vi "260pt Mov Avg.vi"(10 "Value in":dbl) -> (2 "Value out":dbl)   [LabVIEW 2014]
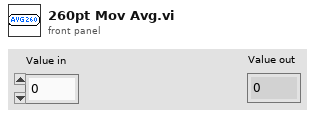
[diagram p1: front panel]
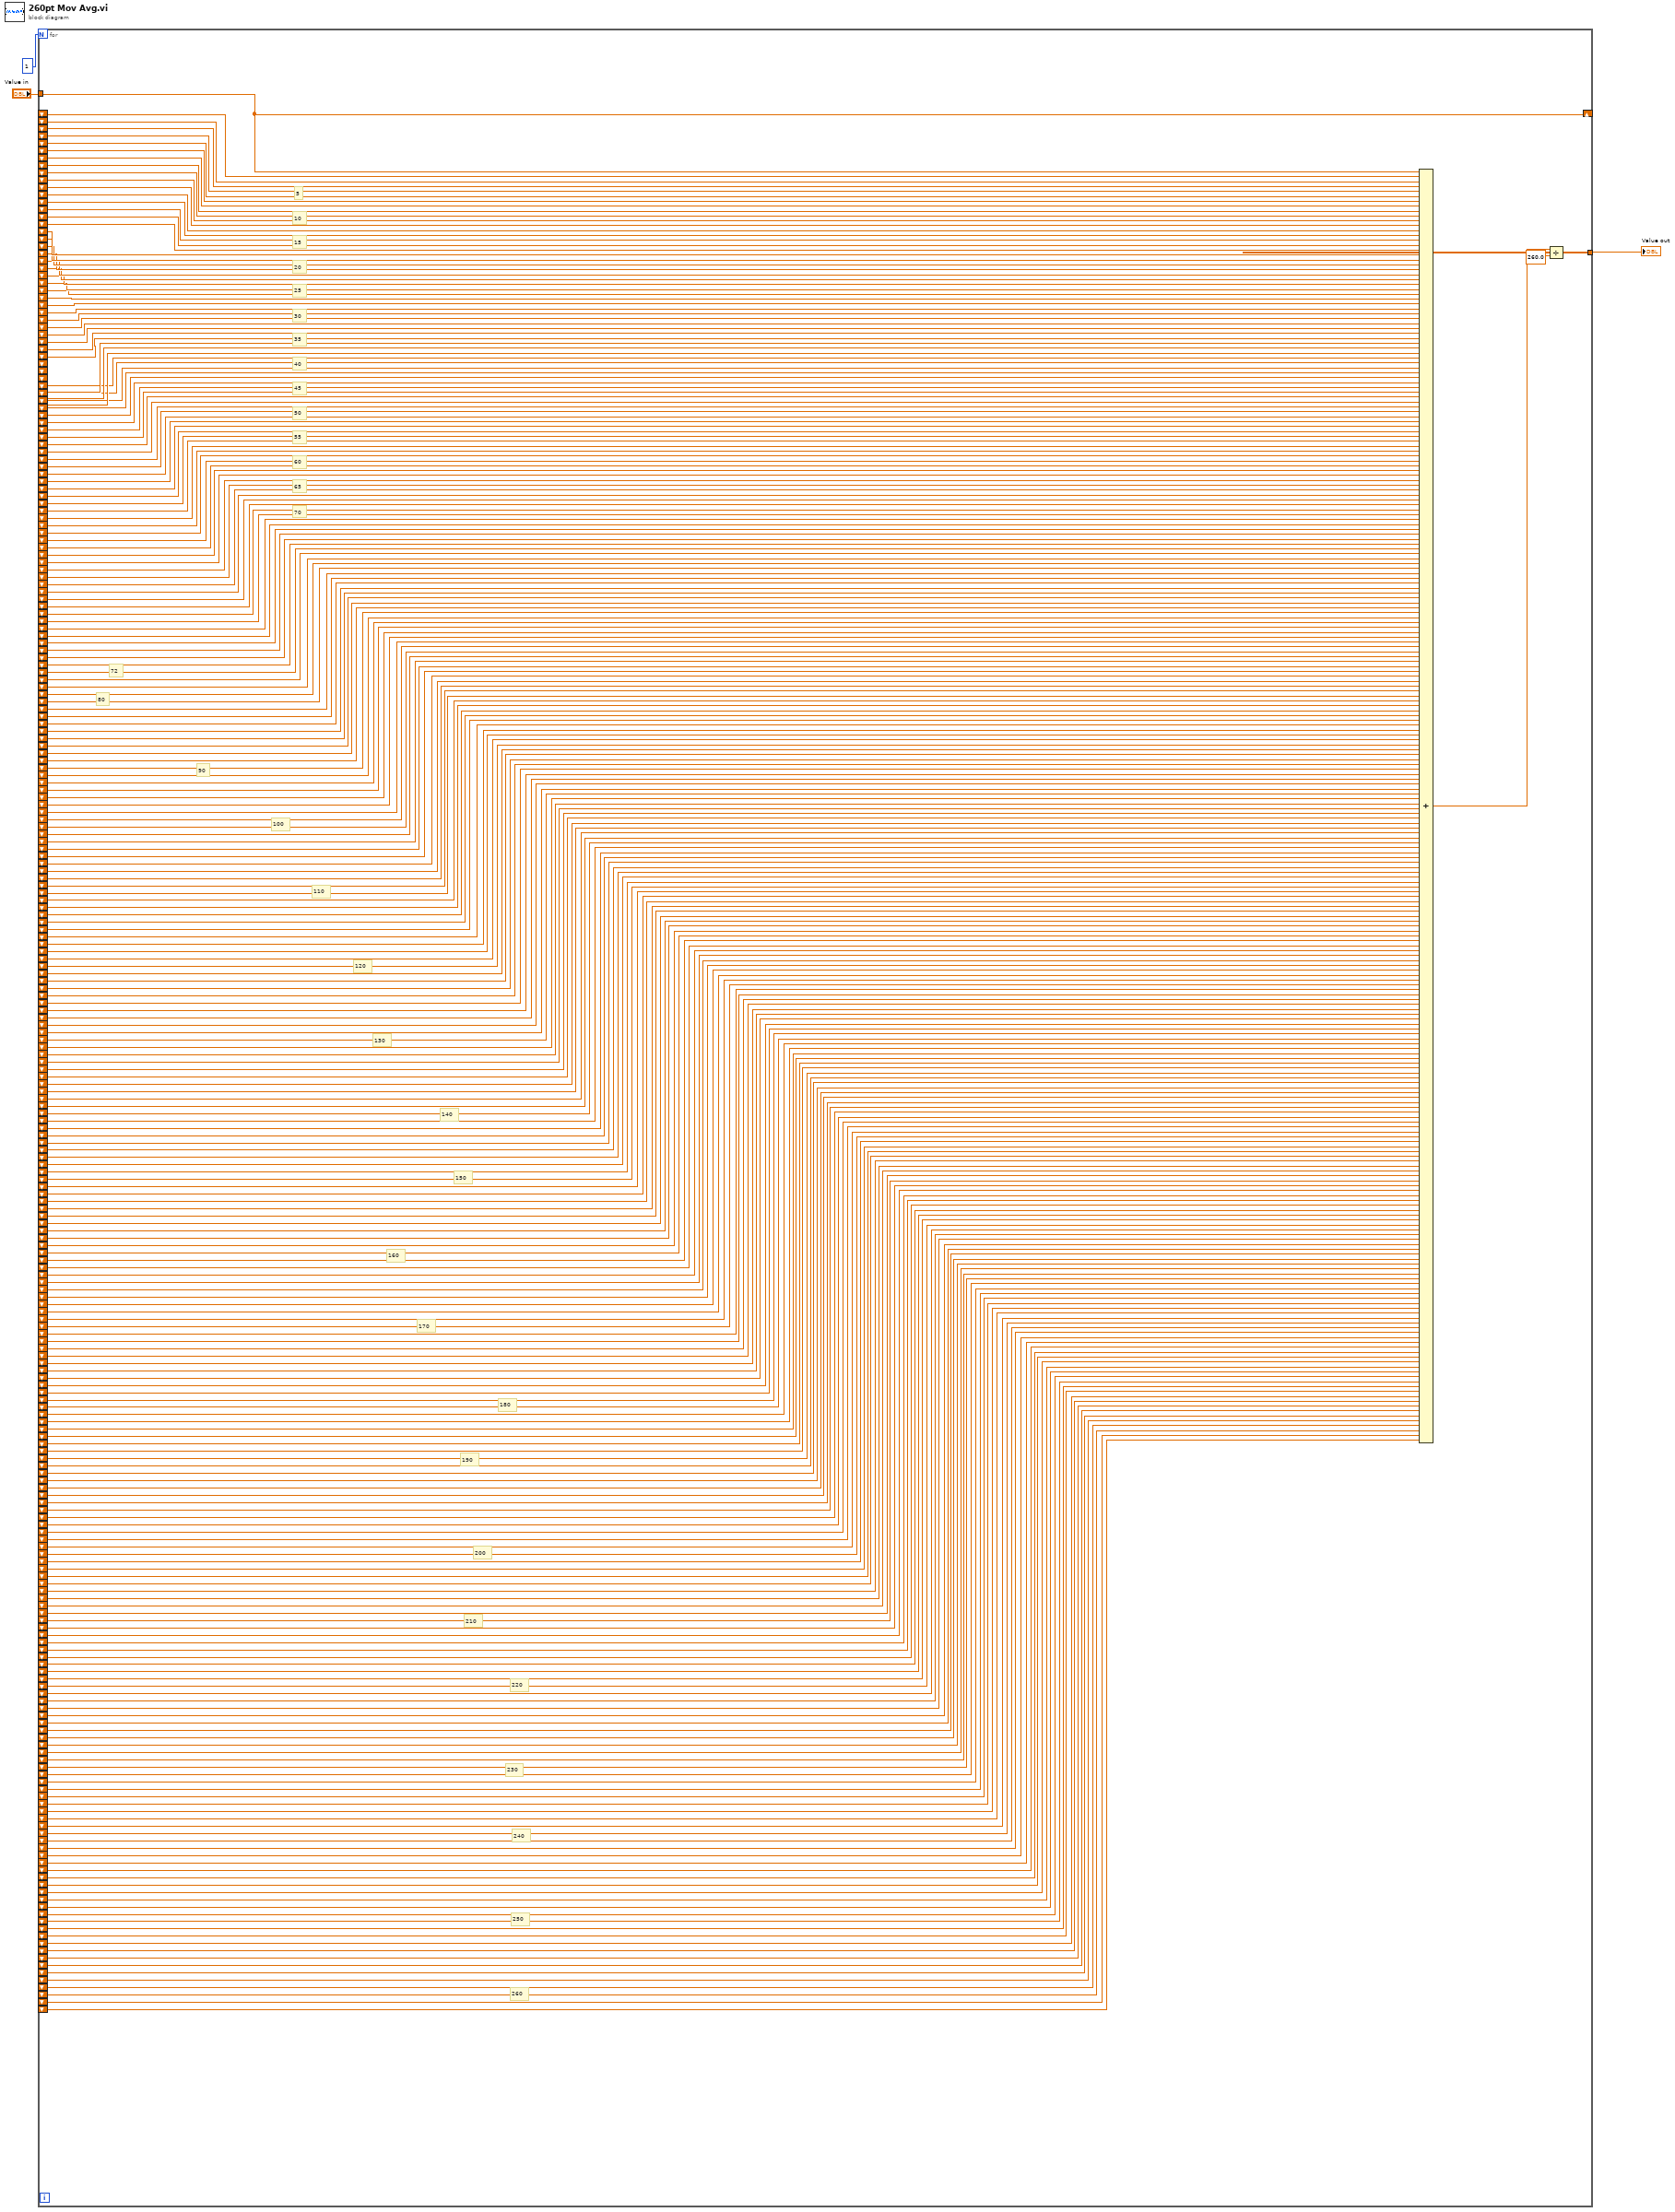
[diagram p0: block diagram]
diagram:
  n1 = for {
    N: 1 -> [_]
    tunnel: "Value in" -> [w266]
    shift-right: [w266] -> _
    shift-left: _ -> [w265]
    shift-left: _ -> [w264]
    shift-left: _ -> [w263]
    shift-left: _ -> [w262]
    tunnel: [w259] -> w1
    shift-left: _ -> [w258]
    shift-left: _ -> [w257]
    shift-left: _ -> [w256]
    shift-left: _ -> [w255]
    shift-left: _ -> [w254]
    shift-left: _ -> [w253]
    shift-left: _ -> [w252]
    shift-left: _ -> [w251]
    shift-left: _ -> [w250]
    shift-left: _ -> [w249]
    shift-left: _ -> [w248]
    shift-left: _ -> [w247]
    shift-left: _ -> [w246]
    shift-left: _ -> [w245]
    shift-left: _ -> [w244]
    shift-left: _ -> [w243]
    shift-left: _ -> [w242]
    shift-left: _ -> [w241]
    shift-left: _ -> [w240]
    shift-left: _ -> [w239]
    shift-left: _ -> [w238]
    shift-left: _ -> [w237]
    shift-left: _ -> [w236]
    shift-left: _ -> [w235]
    shift-left: _ -> [w234]
    shift-left: _ -> [w233]
    shift-left: _ -> [w232]
    shift-left: _ -> [w231]
    shift-left: _ -> [w230]
    shift-left: _ -> [w229]
    shift-left: _ -> [w228]
    shift-left: _ -> [w227]
    shift-left: _ -> [w226]
    shift-left: _ -> [w225]
    shift-left: _ -> [w223]
    shift-left: _ -> [w224]
    shift-left: _ -> [w222]
    shift-left: _ -> [w221]
    shift-left: _ -> [w220]
    shift-left: _ -> [w219]
    shift-left: _ -> [w218]
    shift-left: _ -> [w217]
    shift-left: _ -> [w216]
    shift-left: _ -> [w215]
    shift-left: _ -> [w214]
    shift-left: _ -> [w213]
    shift-left: _ -> [w212]
    shift-left: _ -> [w211]
    shift-left: _ -> [w210]
    shift-left: _ -> [w209]
    shift-left: _ -> [w208]
    shift-left: _ -> [w207]
    shift-left: _ -> [w206]
    shift-left: _ -> [w205]
    shift-left: _ -> [w204]
    shift-left: _ -> [w203]
    shift-left: _ -> [w202]
    shift-left: _ -> [w201]
    shift-left: _ -> [w200]
    shift-left: _ -> [w199]
    shift-left: _ -> [w198]
    shift-left: _ -> [w197]
    shift-left: _ -> [w196]
    shift-left: _ -> [w195]
    shift-left: _ -> [w194]
    shift-left: _ -> [w193]
    shift-left: _ -> [w192]
    shift-left: _ -> [w191]
    shift-left: _ -> [w190]
    shift-left: _ -> [w189]
    shift-left: _ -> [w188]
    shift-left: _ -> [w187]
    shift-left: _ -> [w186]
    shift-left: _ -> [w185]
    shift-left: _ -> [w184]
    shift-left: _ -> [w183]
    shift-left: _ -> [w182]
    shift-left: _ -> [w181]
    shift-left: _ -> [w180]
    shift-left: _ -> [w179]
    shift-left: _ -> [w178]
    shift-left: _ -> [w177]
    shift-left: _ -> [w176]
    shift-left: _ -> [w175]
    shift-left: _ -> [w174]
    shift-left: _ -> [w173]
    shift-left: _ -> [w172]
    shift-left: _ -> [w171]
    shift-left: _ -> [w170]
    shift-left: _ -> [w169]
    shift-left: _ -> [w168]
    shift-left: _ -> [w167]
    shift-left: _ -> [w166]
    shift-left: _ -> [w165]
    shift-left: _ -> [w164]
    shift-left: _ -> [w163]
    shift-left: _ -> [w162]
    shift-left: _ -> [w161]
    shift-left: _ -> [w160]
    shift-left: _ -> [w159]
    shift-left: _ -> [w158]
    shift-left: _ -> [w157]
    shift-left: _ -> [w156]
    shift-left: _ -> [w155]
    shift-left: _ -> [w154]
    shift-left: _ -> [w153]
    shift-left: _ -> [w152]
    shift-left: _ -> [w151]
    shift-left: _ -> [w150]
    shift-left: _ -> [w149]
    shift-left: _ -> [w148]
    shift-left: _ -> [w147]
    shift-left: _ -> [w146]
    shift-left: _ -> [w145]
    shift-left: _ -> [w144]
    shift-left: _ -> [w143]
    shift-left: _ -> [w142]
    shift-left: _ -> [w141]
    shift-left: _ -> [w140]
    shift-left: _ -> [w139]
    shift-left: _ -> [w138]
    shift-left: _ -> [w137]
    shift-left: _ -> [w136]
    shift-left: _ -> [w135]
    shift-left: _ -> [w134]
    shift-left: _ -> [w133]
    shift-left: _ -> [w132]
    shift-left: _ -> [w131]
    shift-left: _ -> [w130]
    shift-left: _ -> [w129]
    shift-left: _ -> [w128]
    shift-left: _ -> [w127]
    shift-left: _ -> [w126]
    shift-left: _ -> [w125]
    shift-left: _ -> [w124]
    shift-left: _ -> [w123]
    shift-left: _ -> [w122]
    shift-left: _ -> [w121]
    shift-left: _ -> [w120]
    shift-left: _ -> [w119]
    shift-left: _ -> [w118]
    shift-left: _ -> [w117]
    shift-left: _ -> [w116]
    shift-left: _ -> [w115]
    shift-left: _ -> [w114]
    shift-left: _ -> [w113]
    shift-left: _ -> [w112]
    shift-left: _ -> [w111]
    shift-left: _ -> [w110]
    shift-left: _ -> [w109]
    shift-left: _ -> [w108]
    shift-left: _ -> [w107]
    shift-left: _ -> [w106]
    shift-left: _ -> [w105]
    shift-left: _ -> [w104]
    shift-left: _ -> [w103]
    shift-left: _ -> [w102]
    shift-left: _ -> [w101]
    shift-left: _ -> [w100]
    shift-left: _ -> [w99]
    shift-left: _ -> [w98]
    shift-left: _ -> [w97]
    shift-left: _ -> [w96]
    shift-left: _ -> [w95]
    shift-left: _ -> [w94]
    shift-left: _ -> [w93]
    shift-left: _ -> [w92]
    shift-left: _ -> [w91]
    shift-left: _ -> [w90]
    shift-left: _ -> [w89]
    shift-left: _ -> [w88]
    shift-left: _ -> [w87]
    shift-left: _ -> [w86]
    shift-left: _ -> [w85]
    shift-left: _ -> [w84]
    shift-left: _ -> [w83]
    shift-left: _ -> [w82]
    shift-left: _ -> [w81]
    shift-left: _ -> [w80]
    shift-left: _ -> [w79]
    shift-left: _ -> [w78]
    shift-left: _ -> [w77]
    shift-left: _ -> [w76]
    shift-left: _ -> [w75]
    shift-left: _ -> [w74]
    shift-left: _ -> [w73]
    shift-left: _ -> [w72]
    shift-left: _ -> [w71]
    shift-left: _ -> [w70]
    shift-left: _ -> [w69]
    shift-left: _ -> [w68]
    shift-left: _ -> [w67]
    shift-left: _ -> [w66]
    shift-left: _ -> [w65]
    shift-left: _ -> [w64]
    shift-left: _ -> [w63]
    shift-left: _ -> [w62]
    shift-left: _ -> [w61]
    shift-left: _ -> [w60]
    shift-left: _ -> [w59]
    shift-left: _ -> [w58]
    shift-left: _ -> [w57]
    shift-left: _ -> [w56]
    shift-left: _ -> [w55]
    shift-left: _ -> [w54]
    shift-left: _ -> [w53]
    shift-left: _ -> [w52]
    shift-left: _ -> [w51]
    shift-left: _ -> [w50]
    shift-left: _ -> [w49]
    shift-left: _ -> [w48]
    shift-left: _ -> [w47]
    shift-left: _ -> [w46]
    shift-left: _ -> [w45]
    shift-left: _ -> [w44]
    shift-left: _ -> [w43]
    shift-left: _ -> [w42]
    shift-left: _ -> [w41]
    shift-left: _ -> [w40]
    shift-left: _ -> [w39]
    shift-left: _ -> [w38]
    shift-left: _ -> [w37]
    shift-left: _ -> [w36]
    shift-left: _ -> [w35]
    shift-left: _ -> [w34]
    shift-left: _ -> [w33]
    shift-left: _ -> [w32]
    shift-left: _ -> [w31]
    shift-left: _ -> [w30]
    shift-left: _ -> [w29]
    shift-left: _ -> [w28]
    shift-left: _ -> [w27]
    shift-left: _ -> [w26]
    shift-left: _ -> [w25]
    shift-left: _ -> [w24]
    shift-left: _ -> [w23]
    shift-left: _ -> [w22]
    shift-left: _ -> [w21]
    shift-left: _ -> [w20]
    shift-left: _ -> [w19]
    shift-left: _ -> [w18]
    shift-left: _ -> [w17]
    shift-left: _ -> [w16]
    shift-left: _ -> [w15]
    shift-left: _ -> [w14]
    shift-left: _ -> [w13]
    shift-left: _ -> [w12]
    shift-left: _ -> [w11]
    shift-left: _ -> [w10]
    shift-left: _ -> [w9]
    shift-left: _ -> [w8]
    shift-left: _ -> [w7]
    shift-left: _ -> [w6]
    shift-left: _ -> [w5]
    shift-left: _ -> [w4]
    # "260"
    # "250"
    # "240"
    # "230"
    # "220"
    # "210"
    # "200"
    # "190"
    # "180"
    # "170"
    # "160"
    # "150"
    # "140"
    # "130"
    # "120"
    # "110"
    # "100"
    # "90"
    # "80"
    # "72"
    # "70"
    # "65"
    # "55"
    # "45"
    # "35"
    # "30"
    # "25"
    # "20"
    # "15"
    # "10"
    # "5"
    # "60"
    # "50"
    # "40"
    n2 = Compound Arithmetic op=ADD(w266, w265, w264, w263, w262, w258, w257, w256, w255, w254, w253, w252, w251, w250, w249, w248, w247, w246, w245, w244, w243, w242, w241, w240, w239, w238, w237, w236, w235, w234, w233, w232, w231, w230, w229, w228, w227, w226, w225, w223, w224, w222, w221, w220, w219, w218, w217, w216, w215, w214, w213, w212, w211, w210, w209, w208, w207, w206, w205, w204, w203, w202, w201, w200, w199, w198, w197, w196, w195, w194, w193, w192, w191, w190, w189, w188, w187, w186, w185, w184, w183, w182, w181, w180, w179, w178, w177, w176, w175, w174, w173, w172, w171, w170, w169, w168, w167, w166, w165, w164, w163, w162, w161, w160, w159, w158, w157, w156, w155, w154, w153, w152, w151, w150, w149, w148, w147, w146, w145, w144, w143, w142, w141, w140, w139, w138, w137, w136, w135, w134, w133, w132, w131, w130, w129, w128, w127, w126, w125, w124, w123, w122, w121, w120, w119, w118, w117, w116, w115, w114, w113, w112, w111, w110, w109, w108, w107, w106, w105, w104, w103, w102, w101, w100, w99, w98, w97, w96, w95, w94, w93, w92, w91, w90, w89, w88, w87, w86, w85, w84, w83, w82, w81, w80, w79, w78, w77, w76, w75, w74, w73, w72, w71, w70, w69, w68, w67, w66, w65, w64, w63, w62, w61, w60, w59, w58, w57, w56, w55, w54, w53, w52, w51, w50, w49, w48, w47, w46, w45, w44, w43, w42, w41, w40, w39, w38, w37, w36, w35, w34, w33, w32, w31, w30, w29, w28, w27, w26, w25, w24, w23, w22, w21, w20, w19, w18, w17, w16, w15, w14, w13, w12, w11, w10, w9, w8, w7, w6, w5, w4) -> (w261:dbl)
    n3 = Divide(x=w261, y=260.0) -> (x/y=w259:dbl)
  }
  "Value out" <- w1
